vi "ziModGetHeader.vi"   [LabVIEW 2016, in "Zurich Instruments LabOne.lvlib"]
uses:
  Zurich Instruments LabOne.lvlib
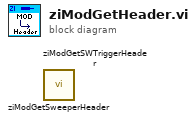
[diagram p0: block diagram]
diagram:
  n1 = call "ziModGetSweeperHeader.vi"() -> ()  [unwired: 9 in, 3 out]
  n2 = call "ziModGetSWTriggerHeader.vi"() -> ()  [unwired: 9 in, 3 out]
